vi "Testing_dll.vi"() -> ()   [LabVIEW 2014, in "Driver_interaction.lvlib" / "Dali_usb_tridonics.lvclass"]
uses:
  Dali_usb_tridonics.lvclass
  Vendor/Dali_usb.lvlib
panel:
  out "close response":i32
  out "close failstring":string
  out "command failstring":string
  out "open failstring":string
  out "response_command":i32
  in  "Address":u16
  in  "command_data":u32
  in  "command":u32
  out "closed":bool
  out "ok":bool
  out "opened":bool
  out "device_handle":i32
  out "Bus version":string
  out "DLL version":string
  out "error out":errorcluster
  in  "error in (no error)":errorcluster
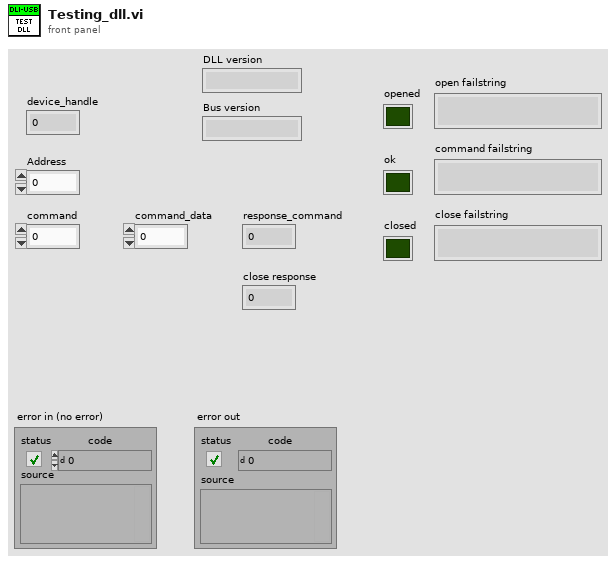
[diagram p1: front panel]
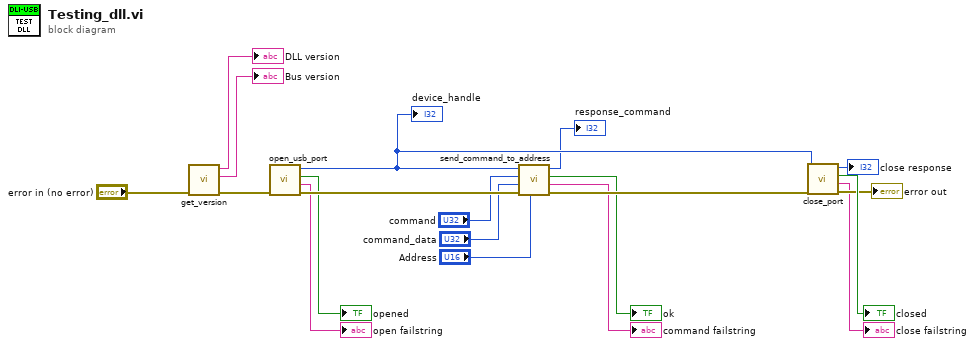
[diagram p0: block diagram]
diagram:
  n1 = call "get_version.vi"("error in (no error)"="error in (no error)") -> ("error out"=w16:errorcluster, "Bus version"=→"Bus version":string, "DLL version"=→"DLL version":string)  [unwired: 8 in]
  n2 = call "open_usb_port.vi"("error in (no error)"=w16) -> ("error out"=w15:errorcluster, "failstring"=→"open failstring":string, "opened"=→"opened":bool, "device_handle"=w19:i32)  [unwired: 7 in]
  "device_handle" <- w19
  n3 = call "send_command_to_address.vi"("Address"="Address", "error in (no error)"=w15, "command_data"="command_data", "command"="command", "device_handle"=w19) -> ("error out"=w14:errorcluster, "failstring"=→"command failstring":string, "ok"=→"ok":bool, "response_command"=→"response_command":i32)  [unwired: 3 in]
  n4 = call "close_port.vi"("error in (no error)"=w14, "device_handle"=w19) -> ("error out"=→"error out":errorcluster, "failstring"=→"close failstring":string, "closed"=→"closed":bool, "close_response"=→"close response":i32)  [unwired: 6 in]
